vi "PV Clean Column.vi"(10 "Column Number":i32=4, 11 "PV Data in":string[][](array[string])) -> (3 "Clean PV Array":string[](array[string]))   [LabVIEW 2023]
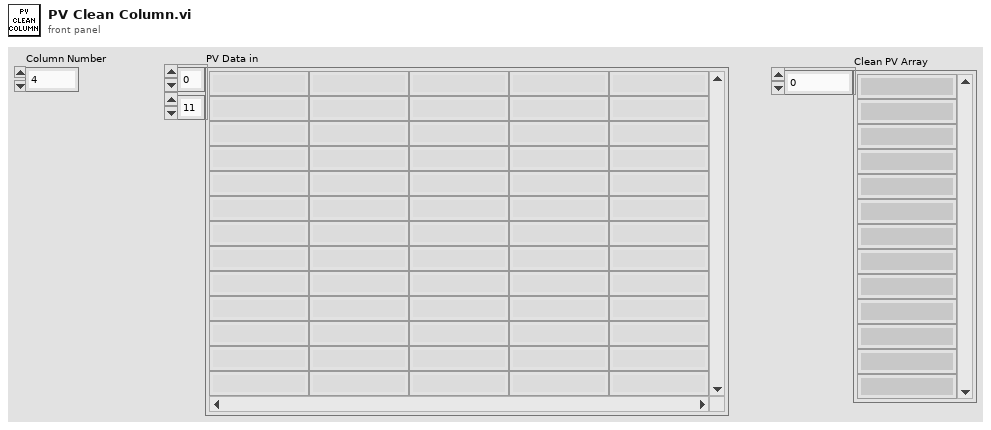
[diagram p1: front panel]
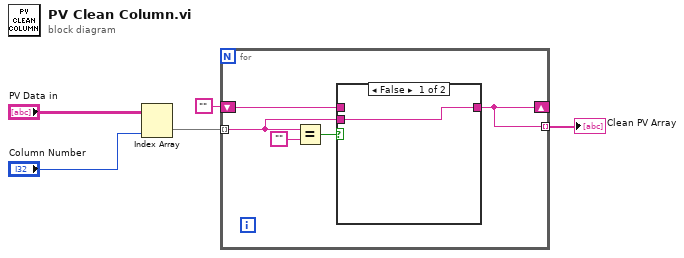
[diagram p0: block diagram]
diagram:
  n1 = Index Array(array="PV Data in", index (col)="Column Number") -> (element=w5:string[])  [unwired: 1 in]
  n2 = for {
    tunnel: w5 -> [w8] mode=indexing
    shift-right: [w6] -> _
    shift-left: "" -> [w7]
    tunnel: [w6] -> w2 mode=indexing
    n3 = Equal?(x=w8, y="") -> (x = y?=w9:bool)
    n4 = case shown="False" w9 {
      tunnel: w8 -> [w11 _]
      tunnel: [w11 w12] -> w6
      tunnel: w7 -> [_ w12]
      frame False {
      }
      frame True {
      }
    }
  }
  "Clean PV Array" <- w2
